vi "COM Increase.vi"(11 "Interface In":refnum<visa-resource-name> caption="通訊位址") -> (3 "Interface Out":refnum<visa-resource-name> caption="通訊位址")   [LabVIEW 2024]
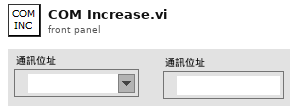
[diagram p1: front panel]
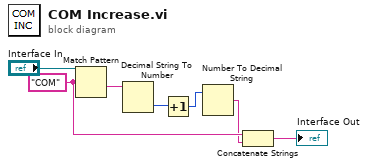
[diagram p0: block diagram]
diagram:
  w3 = "COM" ("regular expression")
  n1 = Match Pattern(string="Interface In", regular expression=w3) -> (after substring=w6:string)  [unwired: 1 in, 3 out]
  n2 = Decimal String To Number(string=w6) -> (number=w5:i32)  [unwired: 2 in, 1 out]
  n3 = Increment(x=w5) -> (x+1=w4:i32)
  n4 = Number To Decimal String(number=w4) -> (decimal integer string=w2:string)  [unwired: 1 in]
  n5 = Concatenate Strings(w3, w2) -> (→"Interface Out":string)
